vi "Create Connection Map From Pin Map File.vi"(8 "error in (no error)":errorcluster, 11 "pin map file path":path) -> (0 "error out":errorcluster, 3 "connection map":map{string, T1[]}(c390))   [LabVIEW 2021, in "PMIC Common.lvlib"]
uses:
  PMIC Common.lvlib
  Instrument Info.ctl
  <vilib>/xml/Load XML File.vi
  <vilib>/xml/Close Reference(Node).vi
  <vilib>/xml/Close Reference(NNMap).vi
  <vilib>/xml/Close Reference(NdList).vi
  <vilib>/xml/NI_XML.lvlib
  <resource>/objmgr/DOMUserDefRef.rc
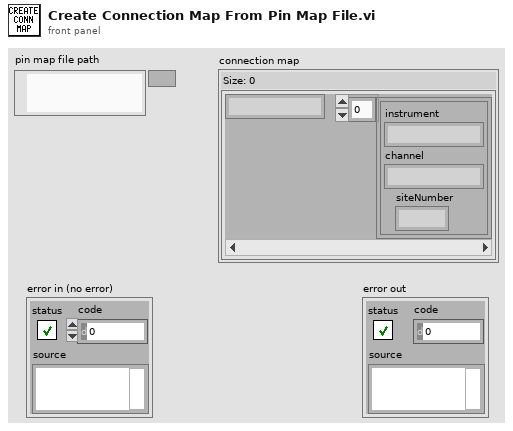
[diagram p1: front panel]
types:
  T1 = typedef "PMIC Common.lvlib/Instrument Info.ctl" = cluster{"instrument":string, "channel":string, "siteNumber":i32}
  T2 = map{string, cluster{"instrument":string, "channel":string, "siteNumber":i32}[]}
  T3 = cluster{"instrument":string, "channel":string, "siteNumber":i32}
  T4 = cluster{"instrument":string, "channel":string, "siteNumber":i32}[]
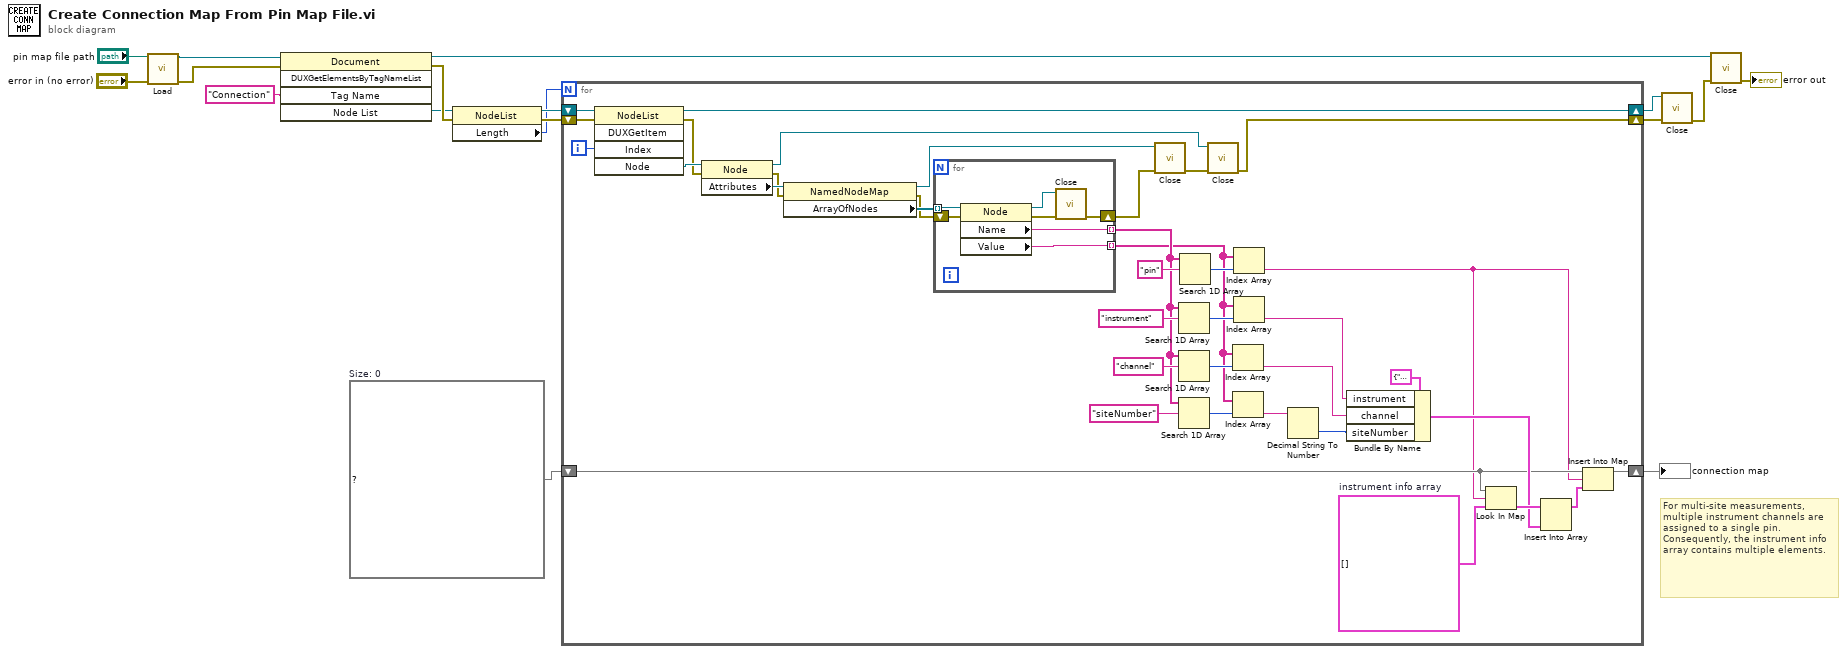
[diagram p0: block diagram]
diagram:
  w3 = T2 {}  # Size: 0
  # "For multi-site measurements, multiple instrument channels are assigned to a single pin. Consequently, the instrument info array contains multiple elements."
  n1 = call-poly <vilib>:"Load.vi"("path to XML document"="pin map file path", "error in (no error)"="error in (no error)") -> ("DOM document out"=w9:refnum<k20>, "error out"=w8:errorcluster)  [unwired: 11 in, 1 out]
  n2 = invoke class="Document" method="DUXGetElementsByTagNameList"(reference=w9, error in=w8, "Tag Name"="Connection") -> (reference out=w16:refnum<k20>, error out=w14:errorcluster, "Node List"=w13:refnum<k20>)  [unwired: 2 in, 2 out]
  n3 = property class="NodeList"(reference=w13, error in=w14) -> (reference out=w12:refnum<k20>, error out=w11:errorcluster, "Length"=w10:i32)
  n4 = for {
    N: w10 -> [_]
    shift-right: [w20] -> w6
    shift-left: w11 -> [w52]
    shift-right: [w26] -> w7
    shift-left: w3 -> [w27]
    shift-right: [w19] -> w5
    shift-left: w12 -> [w53]
    i -> [w51]
    w18 = T4 []  # instrument info array
    n5 = invoke class="NodeList" method="DUXGetItem"(reference=w53, error in=w52, "Index"=w51) -> (reference out=w19:refnum<k20>, error out=w48:errorcluster, "Node"=w54:refnum<k20>)  [unwired: 2 in, 2 out]
    n6 = property class="Node"(reference=w54, error in=w48) -> (reference out=w21:refnum<k20>, error out=w47:errorcluster, "Attributes"=w50:refnum<k20>)
    n7 = property class="NamedNodeMap"(reference=w50, error in=w47) -> (reference out=w23:refnum<k20>, error out=w46:errorcluster, "ArrayOfNodes"=w49:refnum<k20>[])
    n8 = for {
      tunnel: w49 -> [w61] mode=indexing
      tunnel: [w60] -> w37 mode=indexing
      tunnel: [w59] -> w34 mode=indexing
      shift-right: [w55] -> w24
      shift-left: w46 -> [w58]
      n9 = property class="Node"(reference=w61, error in=w58) -> (reference out=w56:refnum<k20>, error out=w57:errorcluster, "Name"=w60:string, "Value"=w59:string)
      n10 = call-poly <vilib>:"Close.vi"("error in (no error)"=w57, "node"=w56) -> ("error out"=w55:errorcluster)  [unwired: 7 in]
    }
    n11 = call-poly <vilib>:"Close.vi"("error in (no error)"=w24, "named node map"=w23) -> ("error out"=w22:errorcluster)  [unwired: 7 in]
    n12 = Search 1D Array(1D array=w37, element="instrument") -> (index of element=w38:i32)  [unwired: 1 in]
    n13 = Search 1D Array(1D array=w37, element="channel") -> (index of element=w36:i32)  [unwired: 1 in]
    n14 = Search 1D Array(1D array=w37, element="siteNumber") -> (index of element=w35:i32)  [unwired: 1 in]
    n15 = Search 1D Array(1D array=w37, element="pin") -> (index of element=w44:i32)  [unwired: 1 in]
    n16 = call-poly <vilib>:"Close.vi"("error in (no error)"=w22, "node"=w21) -> ("error out"=w20:errorcluster)  [unwired: 7 in]
    n17 = Index Array(array=w34, index=w36) -> (element=w31:string)
    n18 = Index Array(array=w34, index=w35) -> (element=w33:string)
    n19 = Index Array(array=w34, index=w44) -> (element=w25:string)
    n20 = Index Array(array=w34, index=w38) -> (element=w30:string)
    n21 = Decimal String To Number(string=w33) -> (number=w32:i32)  [unwired: 2 in, 1 out]
    n22 = Bundle By Name(cluster=T3 {"instrument"="", "channel"="", "siteNumber"=0}, "instrument"=w30, "channel"=w31, "siteNumber"=w32) -> (w29:T3)
    n23 = Look In Map(map=w27, key=w25, default value=w18) -> (value=w43:T4)  [unwired: 1 out]
    n24 = Insert Into Array(array=w43, new element=w29) -> (w28:T4)  [unwired: 1 in]
    n25 = Insert Into Map(map in=w27, key=w25, value=w28) -> (map out=w26:T2)  [unwired: 2 out]
  }
  "connection map" <- w7
  n26 = call-poly <vilib>:"Close.vi"("error in (no error)"=w6, "node list"=w5) -> ("error out"=w4:errorcluster)  [unwired: 7 in]
  n27 = call-poly <vilib>:"Close.vi"("error in (no error)"=w4, "node"=w16) -> ("error out"=→"error out":errorcluster)  [unwired: 7 in]
